vi "getExceptionMessage.vi"(9 "exception":i32, 11 "Job in":refnum<class "Job.lvclass">) -> (0 "exception message":string, 1 "exception dup":i32, 3 "warning?":bool)   [LabVIEW 2013, in "openCronJob.lvlib" / "Job.lvclass"]
uses:
  Job.lvclass
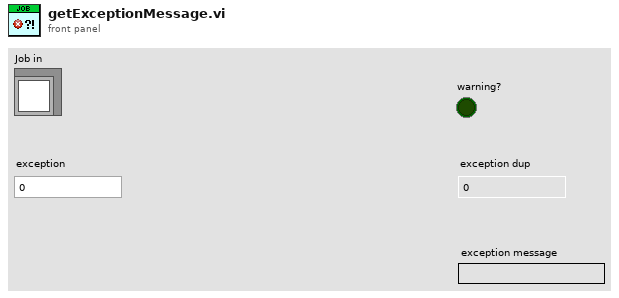
[diagram p1: front panel]
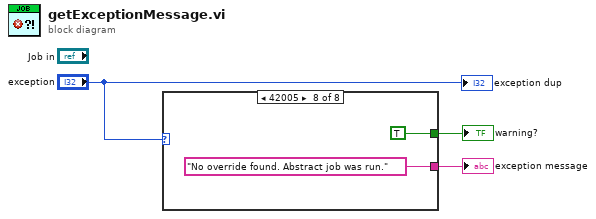
[diagram p0: block diagram]
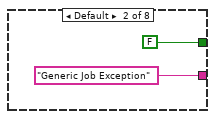
[diagram p3: hidden frame]
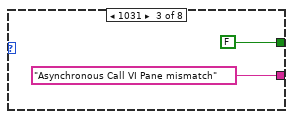
[diagram p4: hidden frame]
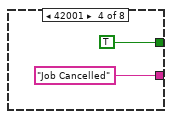
[diagram p5: hidden frame]
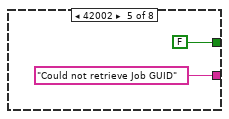
[diagram p6: hidden frame]
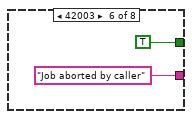
[diagram p7: hidden frame]
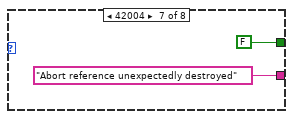
[diagram p8: hidden frame]
diagram:
  n1 = case shown="42005" "exception" {
    tunnel: [_ "Generic Job Exception" ("error message") "Asynchronous Call VI Pane mismatch" ("error message") "Job Cancelled" ("error message") "Could not retrieve Job GUID" ("error message") "Job aborted by caller" ("error message") "Abort reference unexpectedly destroyed" ("error message") "No override found. Abstract job was run." ("error message")] -> w3
    tunnel: [_ FALSE FALSE TRUE FALSE TRUE FALSE TRUE] -> w1
    frame 0 {
    }
    frame Default {
    }
    frame 1031 {
    }
    frame 42001 {
    }
    frame 42002 {
    }
    frame 42003 {
    }
    frame 42004 {
    }
    frame 42005 {
    }
  }
  "exception message" <- w3
  "warning?" <- w1
  "exception dup" <- "exception"
